vi "ScanAction.vi"(8 "error in (no error)":errorcluster caption="entrée d'erreur (pas d'erreur)", 9 "IndicePoint":i32, 10 "Dir":bool, 11 "Tools In":refnum<class "DAQ6363.lvclass"> caption="DNL_LabVIEW Object in") -> (0 "error out":errorcluster caption="sortie d'erreur", 2 "ScanParsOut":dbl[](array[numeric]), 3 "Tools Out":refnum<class "DAQ6363.lvclass"> caption="DNL_LabVIEW Object out")   [LabVIEW 2019, in "DAQ6363.lvclass"]
uses:
  DAQ6363.lvclass
  C:/Programmes Labview/LabscanV1A/DevicesClass/BaseDevice/BaseDevice.lvclass
  DAQ6363.lvclass/DAQ6363.ctl
  <userlib>/GenProg/ReadValByRefTask.vi
  <userlib>/GenProg/ReadValByRefDbl.vi
  <resource>/objmgr/daqmx.rc
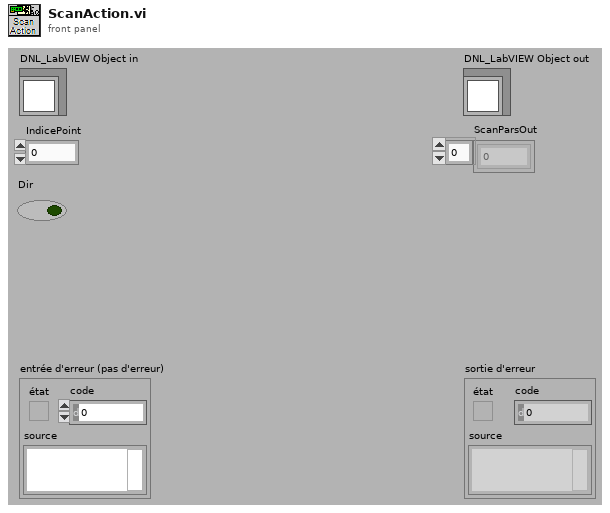
[diagram p1: front panel]
types:
  T1 = typedef "DAQ6363.lvclass/DAQ6363_Func.ctl" = enum16{"CountPulse (Cnt)", "Rabi (Tau)", "MWtoLaserDelay (us)", "APDGate (us)", "PulsedODMR (Pulses)"}
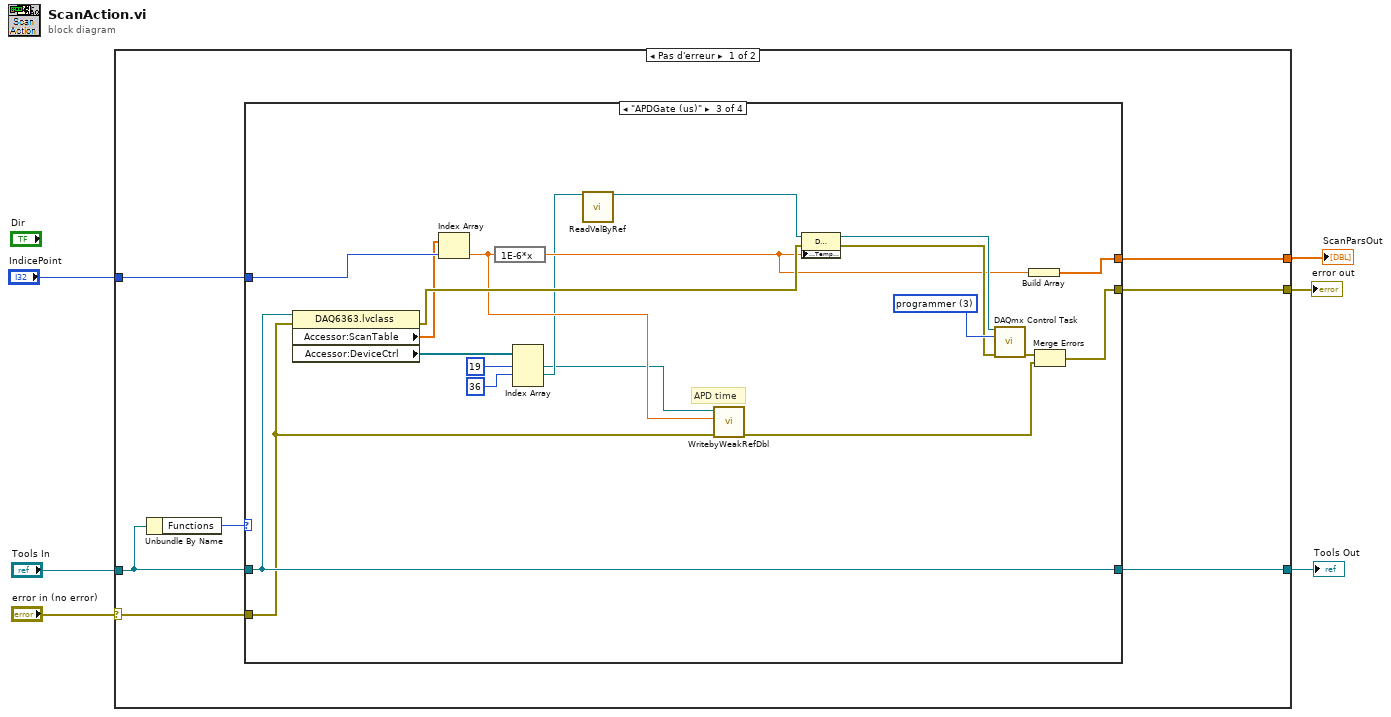
[diagram p0: block diagram]
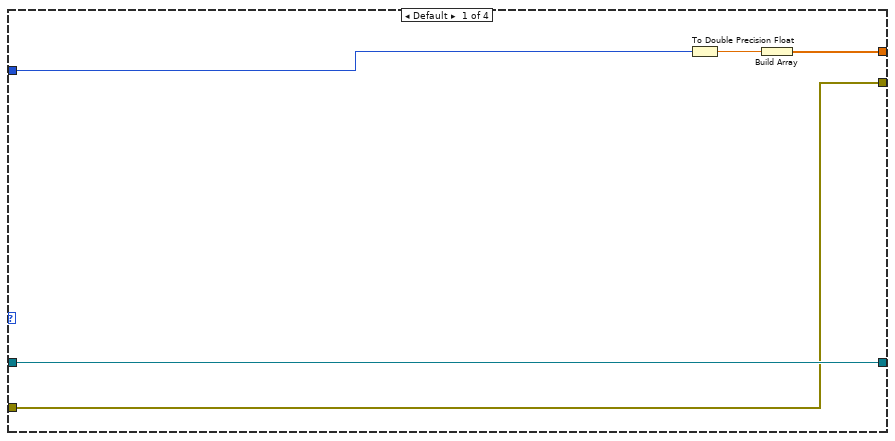
[diagram p2: hidden frame]
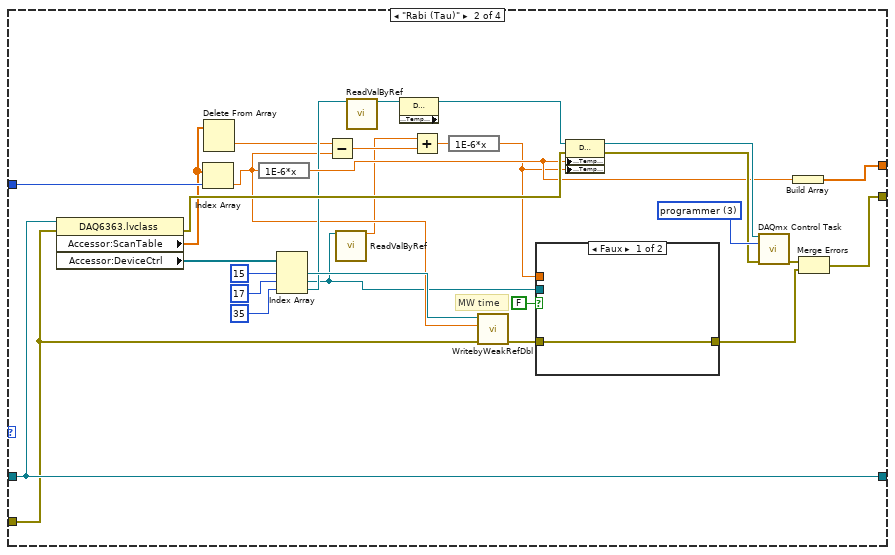
[diagram p3: hidden frame]
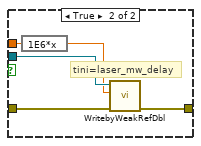
[diagram p4: hidden frame]
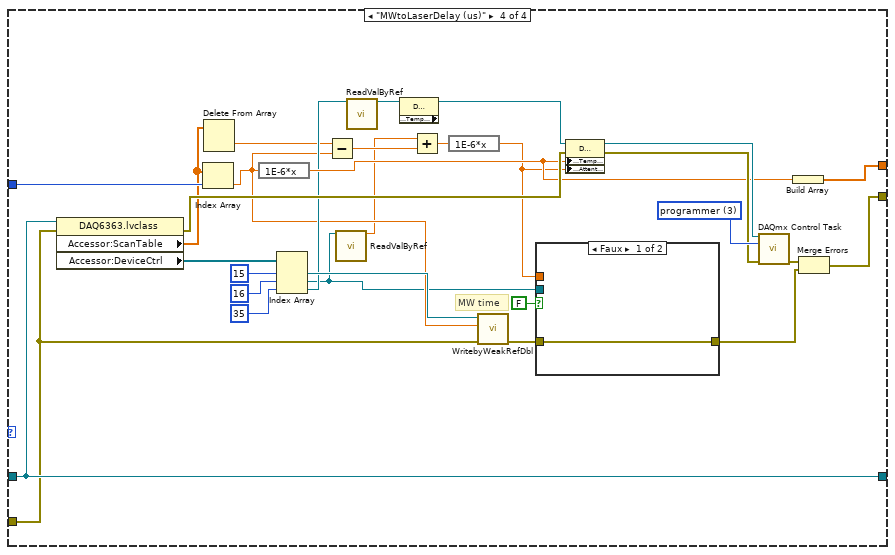
[diagram p5: hidden frame]
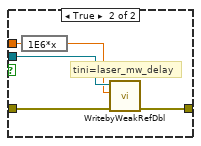
[diagram p6: hidden frame]
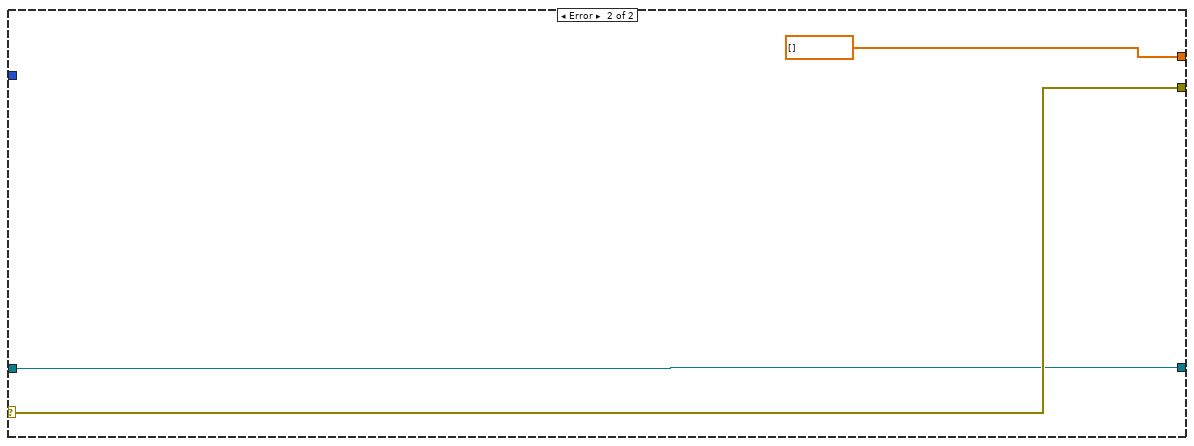
[diagram p7: hidden frame]
diagram:
  n1 = case shown="Pas d'erreur" "error in (no error)" {
    selector: "error in (no error)" -> [w10 w113]
    tunnel: "Tools In" -> [w11 w112]
    tunnel: [w9 dbl[] []] -> w1
    tunnel: [w8 w113] -> w4
    tunnel: [w7 w112] -> w3
    tunnel: "IndicePoint" -> [w12 _]
    frame No Error {
      n2 = Unbundle By Name(w11) -> ("Functions"=w13:T1)
      n3 = case shown="\"APDGate (us)\"" w13 {
        tunnel: [w14 w40 w67 w96] -> w9
        tunnel: w12 -> [w18 w47 w74 w103]
        tunnel: [w16 w38 w65 w94] -> w7
        tunnel: w11 -> [w16 w38 w65 w94]
        tunnel: w10 -> [w15 w29 w62 w85]
        tunnel: [w15 w35 w64 w91] -> w8
        frame Default {
          n4 = To Double Precision Float(number=w18) -> (double precision float=w17:dbl)
          n5 = Build Array(w17) -> (w14:dbl[])
        }
        frame "Rabi (Tau)" {
          w46 = 3 items=["vérifier"=2, "réserver"=4, "programmer"=3, "libérer"=5, "abandonner"=6] ("action")
          # "MW time"
          n6 = property class="DAQ6363.lvclass"(reference=w38, error in=w29) -> (error out=w43:errorcluster, "Accessor:ScanTable"=w28:dbl[], "Accessor:DeviceCtrl"=w30:refnum<vi>[])  [unwired: 1 out]
          n7 = Index Array(array=w28, index=w47) -> (element=w26:dbl)
          n8 = Delete From Array(array=w28) -> (deleted portion=w27:dbl)  [unwired: 2 in, 1 out]
          n9 = expression code="1E-6*x"(w26) -> (w41:dbl)
          n10 = Index Array(array=w30, index #1=15 ("indice"), index #2=17 ("indice"), index #3=35 ("indice")) -> (element #1=w37:refnum<vi>, element #2=w22:refnum<vi>, element #3=w32:refnum<vi>)
          n11 = Subtract(x=w27, y=w26) -> (x-y=w25:dbl)
          n12 = call-poly <userlib>:"ReadValByRef.vi"("Control Ref"=w22) -> ("Valeur"=w20:dbl)  [unwired: 13 in, 1 out]
          n13 = call-poly <userlib>:"ReadValByRef.vi"("Control Ref"=w32) -> ("Valeur"=w33:refnum<k21>)  [unwired: 13 in, 1 out]
          n14 = property class="DAQmx - Voie" props=["CO.Impulsion.TempsBas"](reference=w33) -> (reference out=w48:refnum<k21>)  [unwired: 1 in, 2 out]
          n15 = Add(x=w20, y=w25) -> (x+y=w21:dbl)
          n16 = expression code="1E-6*x"(w21) -> (w24:dbl)
          n17 = call <userlib>:"WritebyWeakRefDbl.vi"("error in"=w29, "Valeur"=w26, "Control Ref"=w37) -> ("error out"=w36:errorcluster)  [unwired: 8 in]
          n18 = case shown="Faux" FALSE {
            tunnel: w22 -> [_ w54]
            tunnel: w36 -> [w49 w52]
            tunnel: [w49 w51] -> w34
            tunnel: w24 -> [_ w50]
            frame False {
            }
            frame True {
              # "tini=laser_mw_delay"
              n19 = expression code="1E6*x"(w50) -> (w53:dbl)
              n20 = call <userlib>:"WritebyWeakRefDbl.vi"("error in"=w52, "Valeur"=w53, "Control Ref"=w54) -> ("error out"=w51:errorcluster)  [unwired: 8 in]
            }
          }
          n21 = property class="DAQmx - Voie"(reference=w48, error in=w43, "CO.Impulsion.TempsHaut"=w41, "CO.Impulsion.TempsBas"=w24) -> (reference out=w45:refnum<k21>, error out=w44:errorcluster)
          n22 = call <vilib>:"DAQmx Control Task.vi"("task/channels in"=w45, "action"=w46, "error in"=w44) -> ("error out"=w42:errorcluster)  [unwired: 11 in, 1 out]
          n23 = Build Array(w41) -> (w40:dbl[])
          n24 = Merge Errors(w42, w34) -> (w35:errorcluster)
        }
        frame "APDGate (us)" {
          w73 = 3 items=["vérifier"=2, "réserver"=4, "programmer"=3, "libérer"=5, "abandonner"=6] ("action")
          # "APD time"
          n25 = property class="DAQ6363.lvclass"(reference=w65, error in=w62) -> (error out=w70:errorcluster, "Accessor:ScanTable"=w61:dbl[], "Accessor:DeviceCtrl"=w63:refnum<vi>[])  [unwired: 1 out]
          n26 = Index Array(array=w61, index=w74) -> (element=w60:dbl)
          n27 = expression code="1E-6*x"(w60) -> (w68:dbl)
          n28 = Index Array(array=w63, index #1=19 ("indice"), index #2=36 ("indice")) -> (element #1=w57:refnum<vi>, element #2=w58:refnum<vi>)  [unwired: 1 in, 1 out]
          n29 = call-poly <userlib>:"ReadValByRef.vi"("Control Ref"=w58) -> ("Valeur"=w55:refnum<k21>)  [unwired: 13 in, 1 out]
          n30 = call <userlib>:"WritebyWeakRefDbl.vi"("error in"=w62, "Valeur"=w60, "Control Ref"=w57) -> ("error out"=w56:errorcluster)  [unwired: 8 in]
          n31 = property class="DAQmx - Voie"(reference=w55, error in=w70, "CO.Impulsion.TempsHaut"=w68) -> (reference out=w72:refnum<k21>, error out=w71:errorcluster)
          n32 = call <vilib>:"DAQmx Control Task.vi"("task/channels in"=w72, "action"=w73, "error in"=w71) -> ("error out"=w69:errorcluster)  [unwired: 11 in, 1 out]
          n33 = Build Array(w68) -> (w67:dbl[])
          n34 = Merge Errors(w69, w56) -> (w64:errorcluster)
        }
        frame "MWtoLaserDelay (us)" {
          w102 = 3 items=["vérifier"=2, "réserver"=4, "programmer"=3, "libérer"=5, "abandonner"=6] ("action")
          # "MW time"
          n35 = property class="DAQ6363.lvclass"(reference=w94, error in=w85) -> (error out=w99:errorcluster, "Accessor:ScanTable"=w84:dbl[], "Accessor:DeviceCtrl"=w86:refnum<vi>[])  [unwired: 1 out]
          n36 = Index Array(array=w84, index=w103) -> (element=w82:dbl)
          n37 = Delete From Array(array=w84) -> (deleted portion=w83:dbl)  [unwired: 2 in, 1 out]
          n38 = expression code="1E-6*x"(w82) -> (w97:dbl)
          n39 = Index Array(array=w86, index #1=15 ("indice"), index #2=16 ("indice"), index #3=35 ("indice")) -> (element #1=w93:refnum<vi>, element #2=w78:refnum<vi>, element #3=w88:refnum<vi>)
          n40 = Subtract(x=w83, y=w82) -> (x-y=w81:dbl)
          n41 = call-poly <userlib>:"ReadValByRef.vi"("Control Ref"=w78) -> ("Valeur"=w76:dbl)  [unwired: 13 in, 1 out]
          n42 = call-poly <userlib>:"ReadValByRef.vi"("Control Ref"=w88) -> ("Valeur"=w89:refnum<k21>)  [unwired: 13 in, 1 out]
          n43 = property class="DAQmx - Voie" props=["CO.Impulsion.TempsBas"](reference=w89) -> (reference out=w104:refnum<k21>)  [unwired: 1 in, 2 out]
          n44 = Add(x=w76, y=w81) -> (x+y=w77:dbl)
          n45 = expression code="1E-6*x"(w77) -> (w80:dbl)
          n46 = call <userlib>:"WritebyWeakRefDbl.vi"("error in"=w85, "Valeur"=w82, "Control Ref"=w93) -> ("error out"=w92:errorcluster)  [unwired: 8 in]
          n47 = case shown="Faux" FALSE {
            tunnel: w78 -> [_ w110]
            tunnel: w92 -> [w105 w108]
            tunnel: [w105 w107] -> w90
            tunnel: w80 -> [_ w106]
            frame False {
            }
            frame True {
              # "tini=laser_mw_delay"
              n48 = expression code="1E6*x"(w106) -> (w109:dbl)
              n49 = call <userlib>:"WritebyWeakRefDbl.vi"("error in"=w108, "Valeur"=w109, "Control Ref"=w110) -> ("error out"=w107:errorcluster)  [unwired: 8 in]
            }
          }
          n50 = property class="DAQmx - Voie"(reference=w104, error in=w99, "CO.Impulsion.TempsHaut"=w97, "CO.Impulsion.Temps.AttenteInitiale"=w80) -> (reference out=w101:refnum<k21>, error out=w100:errorcluster)
          n51 = call <vilib>:"DAQmx Control Task.vi"("task/channels in"=w101, "action"=w102, "error in"=w100) -> ("error out"=w98:errorcluster)  [unwired: 11 in, 1 out]
          n52 = Build Array(w97) -> (w96:dbl[])
          n53 = Merge Errors(w98, w90) -> (w91:errorcluster)
        }
      }
    }
    frame Error {
    }
  }
  "error out" <- w4
  "Tools Out" <- w3
  "ScanParsOut" <- w1
